vi "EZ-Zone PM - Heater Controller.vi"() -> ()   [LabVIEW 2011]
uses:
  Controls/EZ-ZONE Input Cluster.ctl
  Controls/EZ-ZONE Output Cluster.ctl
panel:
  in  "EZ-ZONE Output Cluster":T1={"Loop Control Mode"=10, "Closed Loop Set Point"=75.0, "Open Loop Set Point"=0.0, "Alarm 1 - High Set Point"=150.0, "Alarm 1 - Low Set Point"=0.0, "Alarm 2 - High Set Point"=150.0, "Alarm 2 - Low Set Point"=0.0, "Alarm 3 - High Set Point"=150.0, "Alarm 3 - Low Set Point"=0.0, "Alarm 4 - High Set Point"=150.0, "Alarm 4 - Low Set Point"=0.0, "Profile Action Request"=61, "Profile Start"=0, "Heat Proportional Band"=14.0, "Cool Proportional Band"=14.0, "Time Integral"=180.0, "Time Derivative"=0.0, "Heat Hysteresis"=2.0, "Cool Hysteresis"=2.0, "Dead Band"=0.0} {"Profile Action Request" items=["None"=61, "Start a Profile"=196, "Start a Step"=89, "Pause"=146, "Resume"=147, "End"=148]; "Loop Control Mode" items=["Off"=62, "Auto (closed loop)"=10, "Manual (open loop)"=54]}
  out "EZ-ZONE Input Cluster":T2={"Device Status"=0, "Analog Input Value 1"=0.0, "Analog Input Value 2"=0.0, "Heat Power"=0.0, "Cool Power"=0.0, "Profile Start"=0, "Current Profile"=0, "Current Step"=0, "Active Set Point"=0.0, "Step Time Remaining"=0, "Analog Input Error 1"=61, "Analog Input Error 2"=61, "Alarm State 1"=61, "Alarm State 2"=61, "Alarm State 3"=61, "Alarm State 4"=61, "Digital Input Status 5"=41, "Digital Input Status 6"=41, "Control Mode Active"=62, "Limit State"=62, "Profile Action Request"=61} {"Profile Action Request" items=["None"=61, "Start a Profile"=196, "Start a Step"=89, "Pause"=146, "Resume"=147, "End"=148]; "Limit State" items=["Off"=62, "None"=61, "Limit High"=51, "Limit Low"=52, "Error"=28]; "Control Mode Active" items=["Off"=62, "Auto"=10, "Manual"=54]; "Digital Input Status 6" items=["Inactive"=41, "Active"=5]; "Digital Input Status 5" items=["Inactive"=41, "Active"=5]; "Alarm State 4" items=["Startup"=88, "None"=61, "Blocked"=12, "Alarm Low"=8, "Alarm High"=7, "Error"=28]; "Alarm State 3" items=["Startup"=88, "None"=61, "Blocked"=12, "Alarm Low"=8, "Alarm High"=7, "Error"=28]; "Alarm State 2" items=["Startup"=88, "None"=61, "Blocked"=12, "Alarm Low"=8, "Alarm High"=7, "Error"=28]; "Alarm State 1" items=["Startup"=88, "None"=61, "Blocked"=12, "Alarm Low"=8, "Alarm High"=7, "Error"=28]; "Analog Input Error 2" items=["None"=61, "Open"=65, "Shorted"=127, "Measurement Error"=140, "Bad Calibration Data"=139, "Ambient Error"=9, "RTD Lead Resistance Error"=141]; "Analog Input Error 1" items=["None"=61, "Open"=65, "Shorted"=127, "Measurement Error"=140, "Bad Calibration Data"=139, "Ambient Error"=9, "RTD Lead Resistance Error"=141]}
  in  "stop":bool
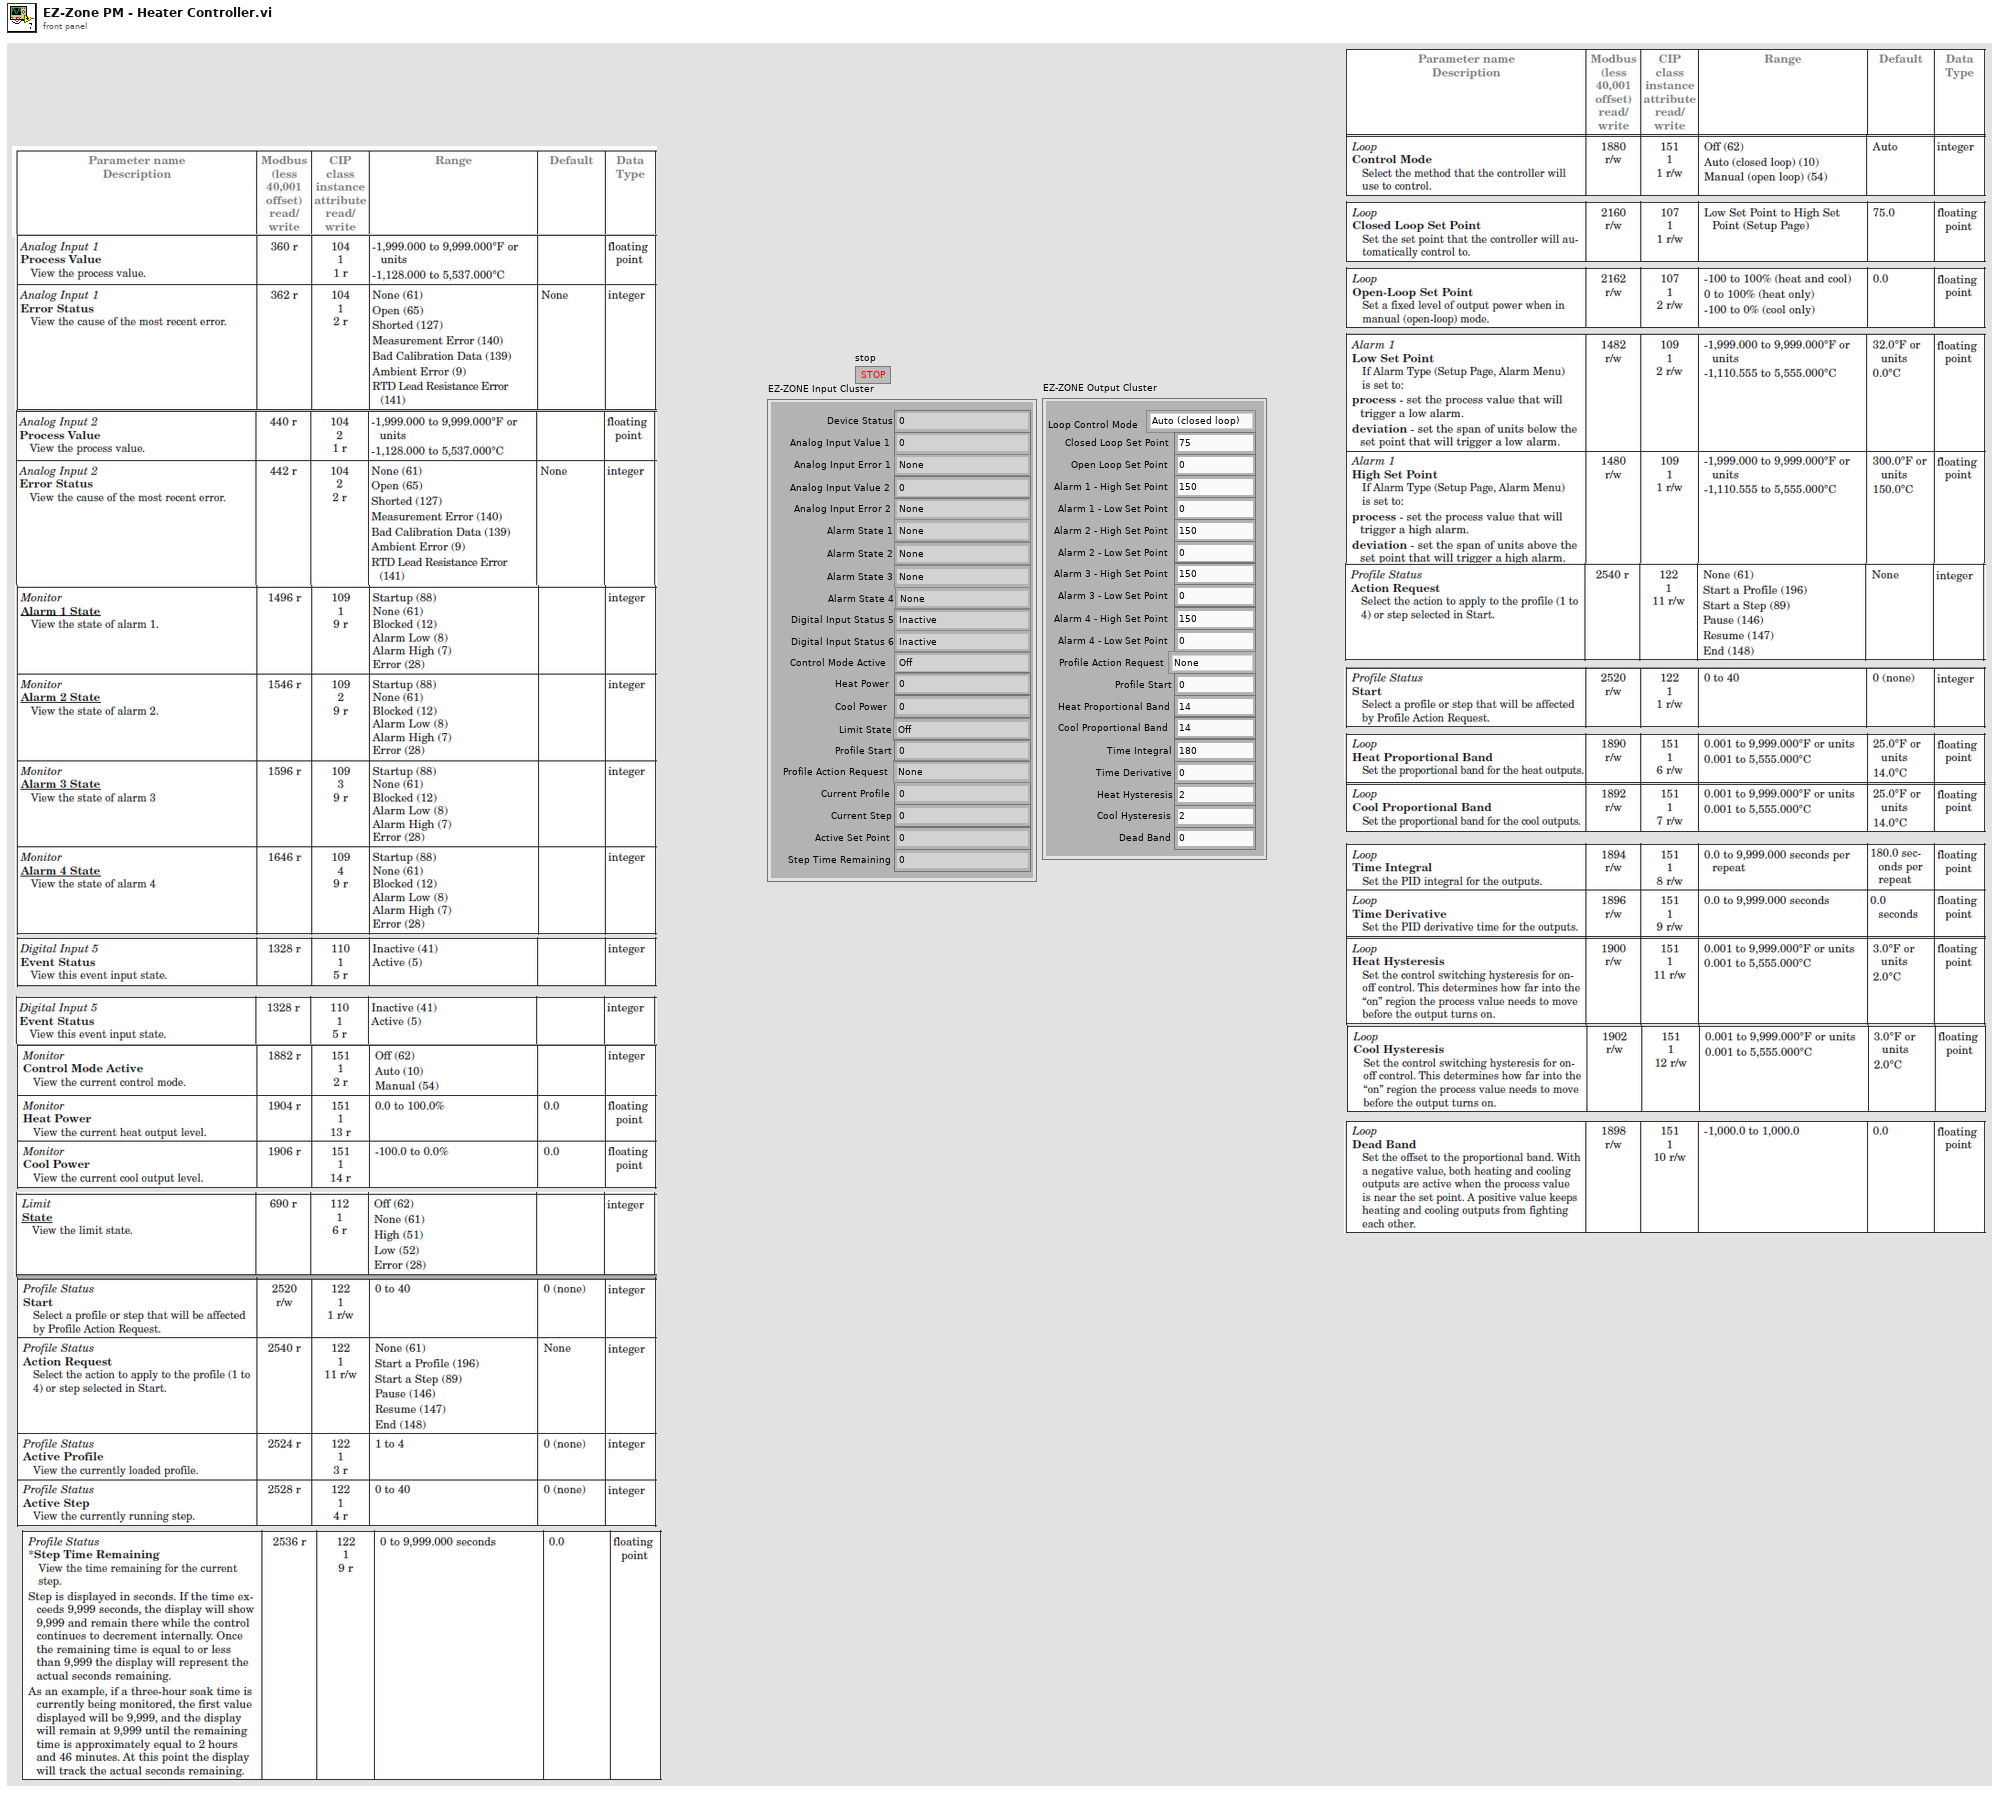
[diagram p1: front panel]
types:
  T1 = typedef "EZ-ZONE Output Cluster.ctl" = cluster{"Loop Control Mode":u32, "Closed Loop Set Point":sgl, "Open Loop Set Point":sgl, "Alarm 1 - High Set Point":sgl, "Alarm 1 - Low Set Point":sgl, "Alarm 2 - High Set Point":sgl, "Alarm 2 - Low Set Point":sgl, "Alarm 3 - High Set Point":sgl, "Alarm 3 - Low Set Point":sgl, "Alarm 4 - High Set Point":sgl, "Alarm 4 - Low Set Point":sgl, "Profile Action Request":u32, "Profile Start":u32, "Heat Proportional Band":sgl, "Cool Proportional Band":sgl, "Time Integral":sgl, "Time Derivative":sgl, "Heat Hysteresis":sgl, "Cool Hysteresis":sgl, "Dead Band":sgl}
  T2 = typedef "EZ-ZONE Input Cluster.ctl" = cluster{"Device Status":u32, "Analog Input Value 1":sgl, "Analog Input Value 2":sgl, "Heat Power":sgl, "Cool Power":sgl, "Profile Start":u32, "Current Profile":u32, "Current Step":u32, "Active Set Point":sgl, "Step Time Remaining":u32, "Analog Input Error 1":u32, "Analog Input Error 2":u32, "Alarm State 1":u32, "Alarm State 2":u32, "Alarm State 3":u32, "Alarm State 4":u32, "Digital Input Status 5":u32, "Digital Input Status 6":u32, "Control Mode Active":u32, "Limit State":u32, "Profile Action Request":u32}
  T3 = enum16{"OPC Server", "Global", "Dnet1", "Dnet2", "Dnet3", "Ain1", "Ain2", "Aout1", "Din1", "Din2", "Dout1"}
  T4 = enum16{"Read", "Write", "ReadWrite", "BufferedRead", "BufferedReadWrite"}
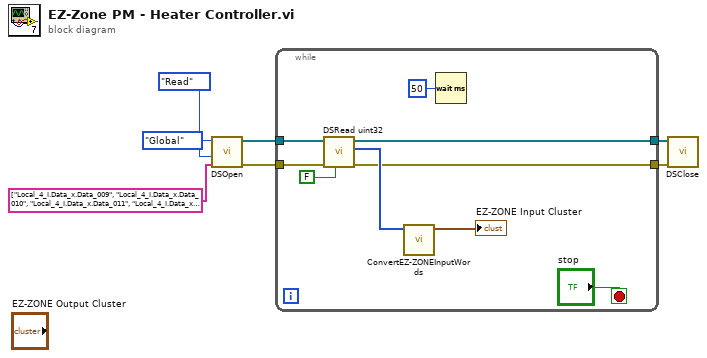
[diagram p0: block diagram]
diagram:
  n1 = call "DSOpen.vi"("Array"=string[] ["Local_4_I.Data_x.Data_009", "Local_4_I.Data_x.Data_010", "Local_4_I.Data_x.Data_011", "Local_4_I.Data_x.Data_012", "Local_4_I.Data_x.Data_013", "Local_4_I.Data_x.Data_014", "Local_4_I.Data_x.Data_015", "Local_4_I.Data_x.Data_016", "Local_4_I.Data_x.Data_017", "Local_4_I.Data_x.Data_018", "Local_4_I.Data_x.Data_019", "Local_4_I.Data_x.Data_020", "Local_4_I.Data_x.Data_021", "Local_4_I.Data_x.Data_022", "Local_4_I.Data_x.Data_023", "Local_4_I.Data_x.Data_024", "Local_4_I.Data_x.Data_025", "Local_4_I.Data_x.Data_026", "Local_4_I.Data_x.Data_027", "Local_4_I.Data_x.Data_028", "Local_4_I.Data_x.Data_029"], "mode"=T4."Read", "Slot"=T3."Global") -> ("error Out"=w7:errorcluster[], "connection out"=w6:refnum<k13>[])  [unwired: 7 in]
  n2 = while {
    tunnel: w7 -> [w15]
    tunnel: w6 -> [w14]
    tunnel: [w13] -> w5
    tunnel: [w12] -> w4
    stop <- "stop" stop-if-true
    n3 = call "DSRead uint32.vi"("wait for updated value (T)"=FALSE, "error in"=w15, "connection in"=w14) -> ("error out"=w13:errorcluster[], "data"=w16:u32[], "connection out"=w12:refnum<k13>[])  [unwired: 6 in]
    n4 = call "ConvertEZ-ZONEInputWords.vi"("Word Array"=w16) -> ("EZ-ZONE Input Cluster"=→"EZ-ZONE Input Cluster":T2)  [unwired: 10 in]
    n5 = Wait (ms)(milliseconds to wait=u32 50) -> ()  [unwired: 1 out]
  }
  n6 = call "DSClose.vi"("error in (no error)"=w5, "connection id"=w4) -> ()  [unwired: 10 in]
